vi "Lower Compress Stop.vi"(8 "error in (no error)":errorcluster, 9 "Motion.lvclass":refnum<class "Motion.lvclass">, 10 "I-O.lvclass":refnum<class "I-O.lvclass">, 11 "Pick and Place in":refnum<class "Pick and Place.lvclass">) -> (0 "error out":errorcluster, 1 "Motion.lvclass":refnum<class "Motion.lvclass">, 2 "I-O out":refnum<class "I-O.lvclass">, 3 "Pick and Place Out":refnum<class "Pick and Place.lvclass">)   [LabVIEW 2016, in "Pick and Place.lvclass"]
uses:
  Pick and Place.lvclass
  Controller/I-O/I-O.lvclass
  Controller/Motion/Motion.lvclass
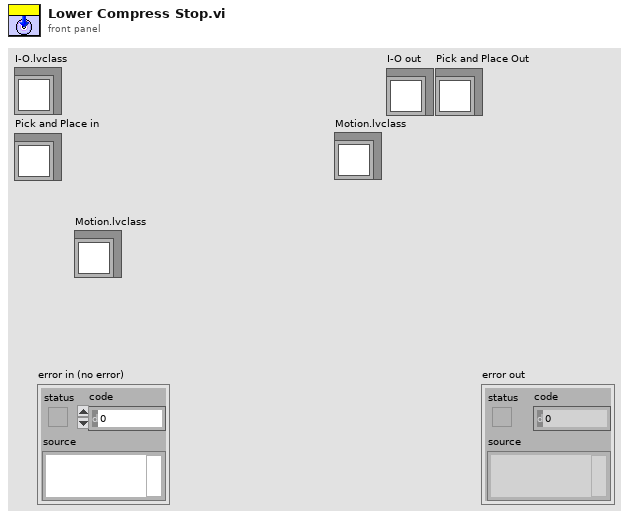
[diagram p1: front panel]
types:
  T1 = typedef "I-O.lvclass/Pin Map.ctl" = cluster{"Region Valves":i32[], "Extra Valves":dbl[][][], "Tool Primary Valve":i32, "Tool Secondary Valve":i32, "Region Sensors":i32[], "Extra Sensors":dbl[][][], "Tool Primary Sensor":dbl, "Tool Secondary Sensor":dbl, "Compression Sensor":dbl, "5V":i32}
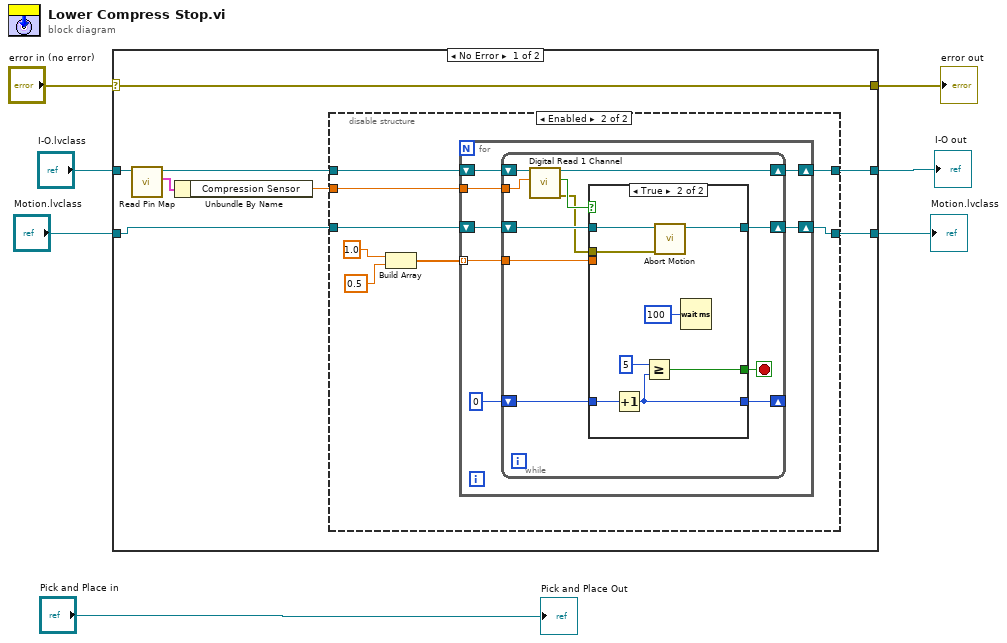
[diagram p0: block diagram]
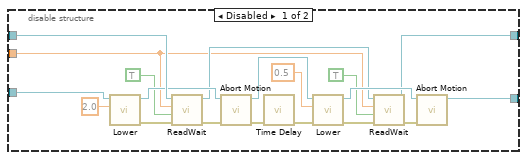
[diagram p2: hidden frame]
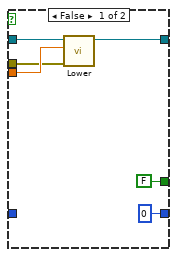
[diagram p3: hidden frame]
diagram:
  n1 = case shown="No Error" "error in (no error)" {
    selector: "error in (no error)" -> [w15 w77]
    tunnel: [w15 w77] -> w6
    tunnel: "I-O.lvclass" -> [w13 w76]
    tunnel: [w8 w76] -> w4
    tunnel: [w9 w75] -> w2
    tunnel: "Motion.lvclass" -> [w14 w75]
    frame No Error {
      n2 = call-dynamic "Read Pin Map.vi"("I-O in"=w13) -> ("Pin Map 2"=w11:T1, "I-O out"=w12:refnum<class "I-O.lvclass">)  [unwired: 8 in, 1 out]
      n3 = Unbundle By Name(w11) -> ("Compression Sensor"=w10:dbl)
      n4 = disable-structure shown="Enabled" {
        disable-tunnel: w14 -> [w32 w36]
        disable-tunnel: w12 -> [w31 w41]
        disable-tunnel: w10 -> [w18 w42]
        disable-tunnel: [w17 w35] -> w9
        disable-tunnel: [w16 w40] -> w8
        frame Disabled {
          n5 = call-dynamic "Lower.vi"("Speed"=2.0, "Motion in"=w32) -> ("error out"=w33:errorcluster, "Motion out"=w30:refnum<class "Motion.lvclass">)  [unwired: 8 in]
          n6 = call "ReadWait.vi"("error in (no error)"=w33, "Value"=TRUE, "Read"=w18, "I-O in"=w31) -> ("error out"=w34:errorcluster, "I-O out"=w20:refnum<class "I-O.lvclass">)  [unwired: 6 in]
          n7 = call-dynamic "Abort Motion.vi"("error in (no error)"=w34, "Motion in"=w30) -> ("error out"=w22:errorcluster, "Motion out"=w19:refnum<class "Motion.lvclass">)  [unwired: 8 in]
          n8 = call "Time Delay"("error in (no error)"=w22) -> ("error out"=w21:errorcluster)  [unwired: 10 in]
          n9 = call-dynamic "Lower.vi"("error in (no error)"=w21, "Speed"=0.5, "Motion in"=w19) -> ("error out"=w26:errorcluster, "Motion out"=w25:refnum<class "Motion.lvclass">)  [unwired: 7 in]
          n10 = call "ReadWait.vi"("error in (no error)"=w26, "Value"=TRUE, "Read"=w18, "I-O in"=w20) -> ("error out"=w27:errorcluster, "I-O out"=w16:refnum<class "I-O.lvclass">)  [unwired: 6 in]
          n11 = call-dynamic "Abort Motion.vi"("error in (no error)"=w27, "Motion in"=w25) -> ("Motion out"=w17:refnum<class "Motion.lvclass">)  [unwired: 8 in, 1 out]
        }
        frame Enabled {
          n12 = Build Array(1.0 ("Speed"), 0.5 ("Speed")) -> (w37:dbl[])
          n13 = for {
            tunnel: w42 -> [w49]
            shift-right: [w47] -> w40
            shift-left: w41 -> [w48]
            tunnel: w37 -> [w45] mode=indexing
            shift-right: [w43] -> w35
            shift-left: w36 -> [w44]
            n14 = while {
              tunnel: w49 -> [w60]
              shift-right: [w58] -> w47
              shift-left: w48 -> [w59]
              shift-right: [w54] -> _
              shift-left: 0 -> [w56]
              tunnel: w45 -> [w53]
              shift-right: [w51] -> w43
              shift-left: w44 -> [w52]
              stop <- w55 stop-if-true
              n15 = call-dynamic "Digital Read 1 Channel.vi"("Read"=w60, "I-O in"=w59) -> ("error out"=w50:errorcluster, "Value"=w57:bool, "I-O out"=w58:refnum<class "I-O.lvclass">)  [unwired: 7 in]
              n16 = case shown="True" w57 {
                tunnel: w56 -> [_ w74]
                tunnel: [FALSE w72] -> w55
                tunnel: [0 w71] -> w54
                tunnel: w53 -> [w64 _]
                tunnel: w52 -> [w63 w69]
                tunnel: [w62 w70] -> w51
                tunnel: w50 -> [w61 w68]
                frame False {
                  n17 = call-dynamic "Lower.vi"("error in (no error)"=w61, "Speed"=w64, "Motion in"=w63) -> ("Motion out"=w62:refnum<class "Motion.lvclass">)  [unwired: 7 in, 1 out]
                }
                frame True {
                  n18 = Increment(x=w74) -> (x+1=w71:i32)
                  n19 = Greater Or Equal?(x=5, y=w71) -> (x >= y?=w72:bool)
                  n20 = call-dynamic "Abort Motion.vi"("error in (no error)"=w68, "Motion in"=w69) -> ("Motion out"=w70:refnum<class "Motion.lvclass">)  [unwired: 8 in, 1 out]
                  n21 = Wait (ms)(milliseconds to wait=u32 100) -> ()  [unwired: 1 out]
                }
              }
            }
          }
        }
      }
    }
    frame Error {
    }
  }
  "error out" <- w6
  "I-O out" <- w4
  "Motion.lvclass" <- w2
  "Pick and Place Out" <- "Pick and Place in"
